vi "Read Factor before collision.vi"(11 "Movable in":refnum<class "Movable.lvclass">) -> (2 "Factor before collision":dbl)   [LabVIEW 2024, in "Movable.lvclass"]
doc: "MIT Licence\nCopyright (c) 2024 David Grollier"
uses:
  Movable.lvclass
  Movable.lvclass/Movable.ctl
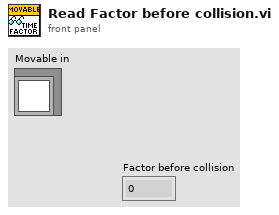
[diagram p1: front panel]
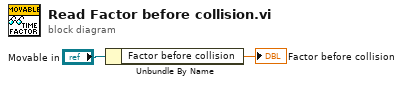
[diagram p0: block diagram]
diagram:
  n1 = Unbundle By Name("Movable in") -> ("Factor before collision"=→"Factor before collision":dbl)
